vi "HGCalSensorTesting.vi"() -> ()   [LabVIEW 2016]
uses:
  <vilib>/Utility/file.llb/Read Delimited Spreadsheet (string).vi
  <vilib>/Utility/file.llb/Read Delimited Spreadsheet (DBL).vi
  <vilib>/Utility/file.llb/Read Delimited Spreadsheet (I64).vi
  <vilib>/Utility/file.llb/Write Delimited Spreadsheet (string).vi
panel:
  in  "Channel to Monitor:":i32
  out "XY Graph 3":cluster{"Y":dbl[], "Y":dbl[]}[](graph)
  in  "Switch Delay (s)":dbl format="%#_13g"
  in  "Voltage Delay (s)":dbl format="%#_13g"
  out "XY Graph 2":cluster{"Y":dbl[], "Y":dbl[]}[](graph)
  out "XY Graph":cluster{"Y":dbl[], "Y":dbl[]}[](graph)
  out "Errors":errorcluster
  in  "Measurement Data":string[][](table)
  in  "Select Measurement Type":enum16{"I-V", "C-V", "Cij"}(ring)
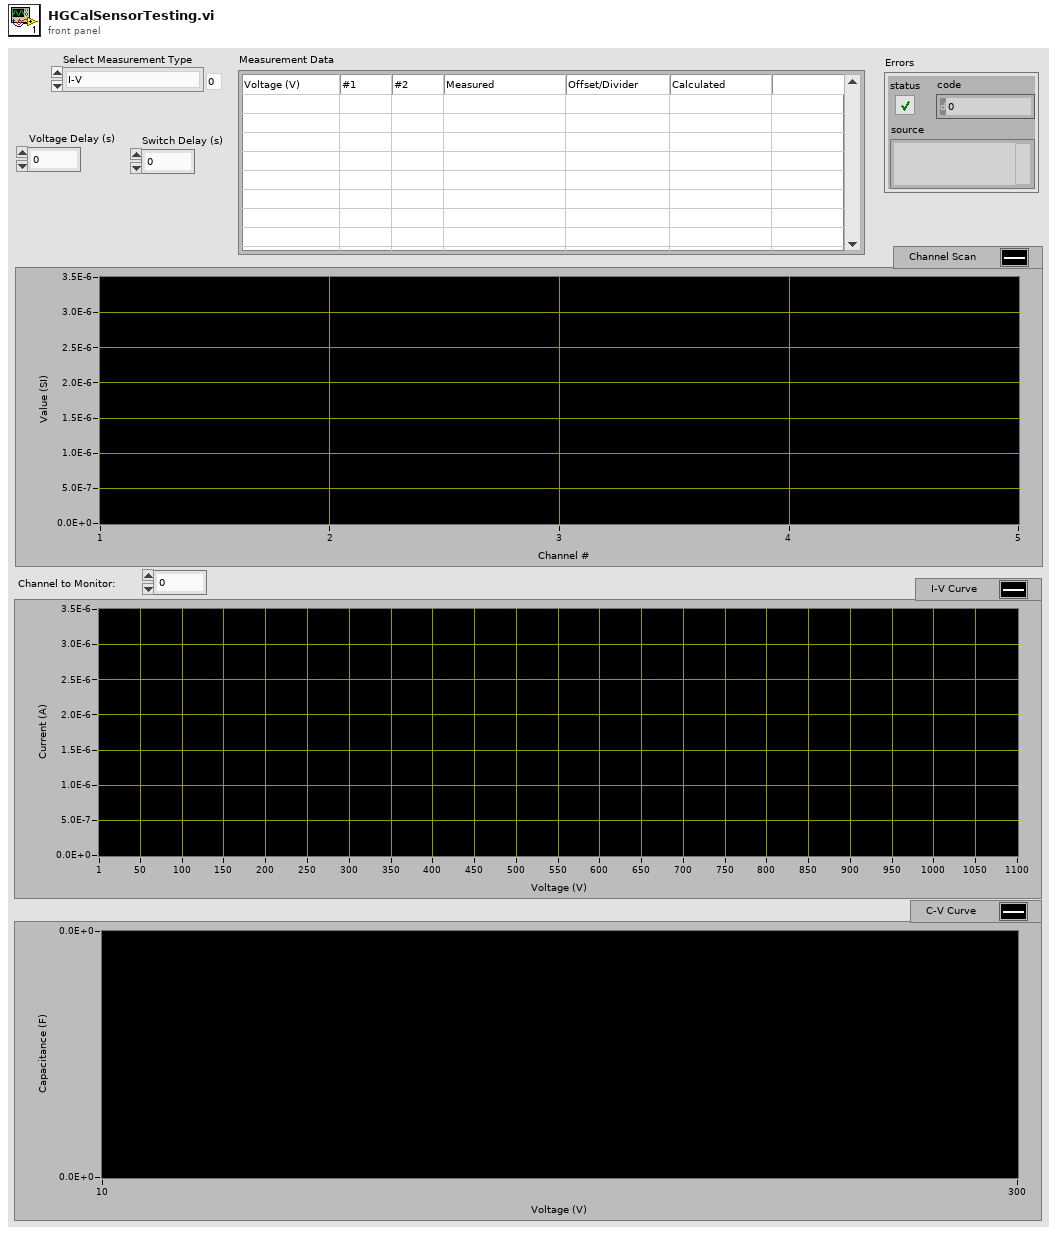
[diagram p1: front panel]
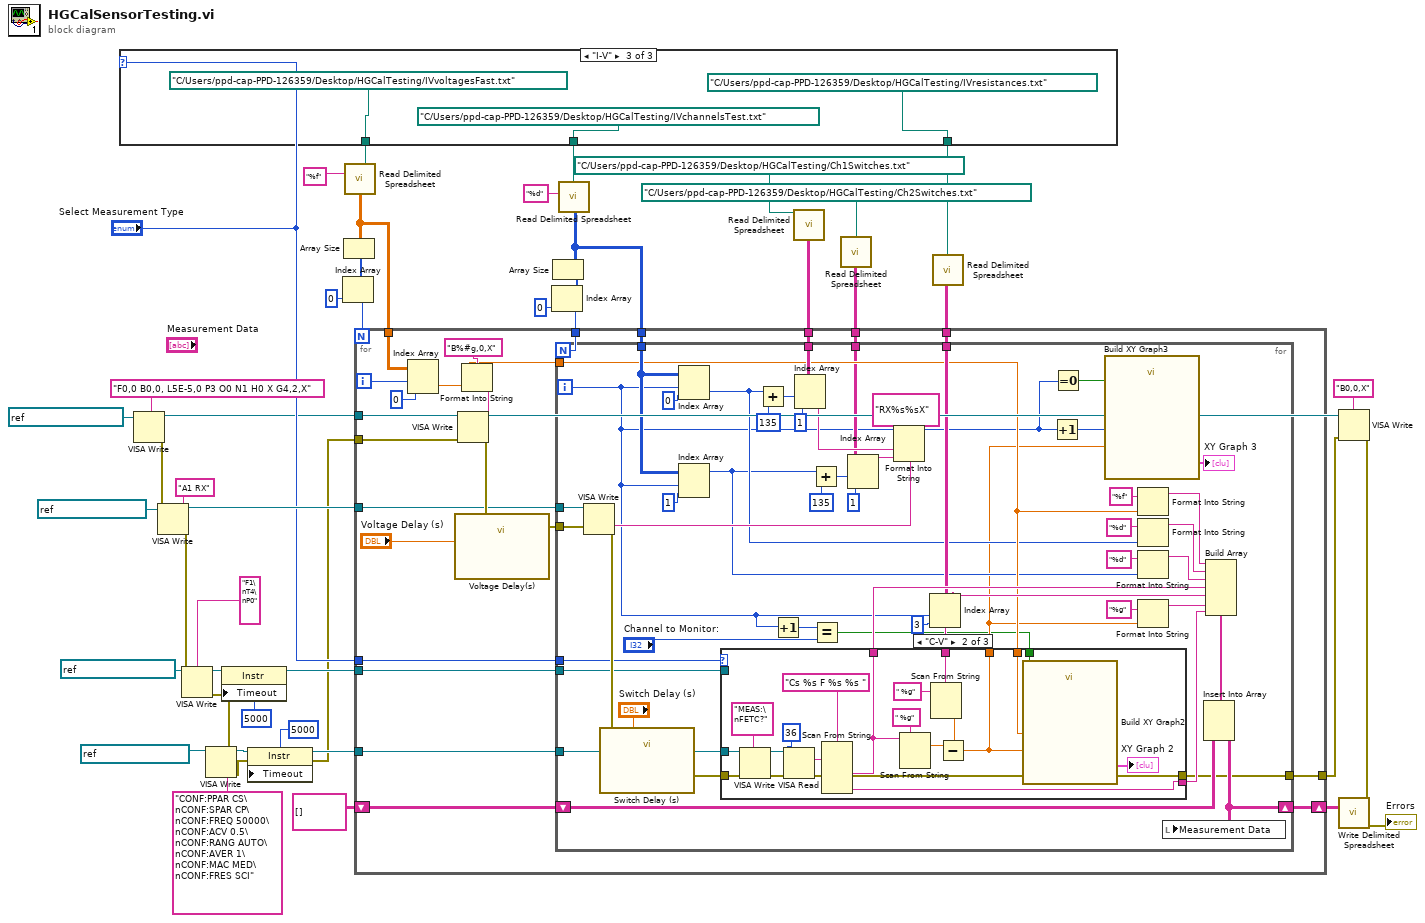
[diagram p0: block diagram]
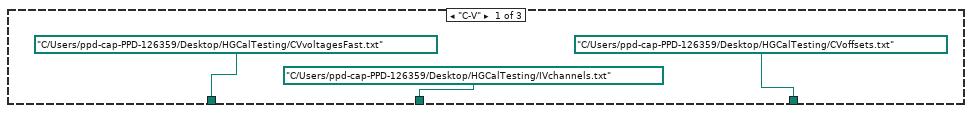
[diagram p2: hidden frame]
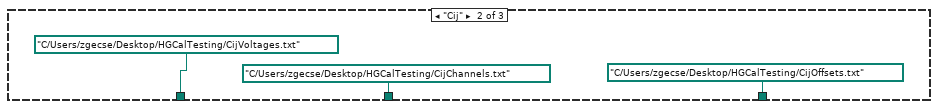
[diagram p3: hidden frame]
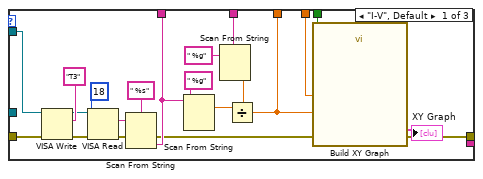
[diagram p4: hidden frame]
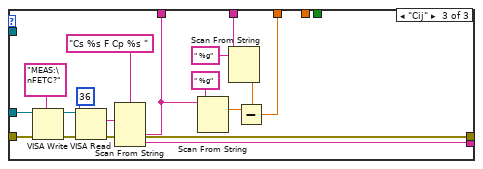
[diagram p5: hidden frame]
diagram:
  n1 = case shown="\"I-V\"" "Select Measurement Type" {
    tunnel: [path "C:/Users/ppd-cap-PPD-126359/Desktop/HGCalTesting/CVvoltagesFast.txt" ("file path (dialog if empty)") path "C:/Users/zgecse/Desktop/HGCalTesting/CijVoltages.txt" ("file path (dialog if empty)") path "C:/Users/ppd-cap-PPD-126359/Desktop/HGCalTesting/IVvoltagesFast.txt" ("file path (dialog if empty)")] -> w37
    tunnel: [path "C:/Users/ppd-cap-PPD-126359/Desktop/HGCalTesting/IVchannels.txt" ("file path (dialog if empty)") path "C:/Users/zgecse/Desktop/HGCalTesting/CijChannels.txt" ("file path (dialog if empty)") path "C:/Users/ppd-cap-PPD-126359/Desktop/HGCalTesting/IVchannelsTest.txt" ("file path (dialog if empty)")] -> w35
    tunnel: [path "C:/Users/ppd-cap-PPD-126359/Desktop/HGCalTesting/CVoffsets.txt" ("file path (dialog if empty)") path "C:/Users/zgecse/Desktop/HGCalTesting/CijOffsets.txt" ("file path (dialog if empty)") path "C:/Users/ppd-cap-PPD-126359/Desktop/HGCalTesting/IVresistances.txt" ("file path (dialog if empty)")] -> w20
    frame "C-V" {
    }
    frame "Cij" {
    }
    frame "I-V" {
    }
  }
  n2 = VISA Write(VISA resource name=refnum<visa-resource-name> "GPIB1::10::INSTR" ("K237 VISA"), write buffer="F0,0 B0,0, L5E-5,0 P3 O0 N1 H0 X G4,2,X" ("F0,0X B%f,0,X L%f,0X P3X O0X")) -> (VISA resource name out=w5:refnum<visa-resource-name>, error out=w43:errorcluster)  [unwired: 1 in, 1 out]
  n3 = VISA Write(VISA resource name=refnum<visa-resource-name> "GPIB1::3::INSTR" ("K706 VISA"), write buffer="A1 RX" ("F0,0X B%f,0,X L%f,0X P3X O0X"), error in (no error)=w43) -> (VISA resource name out=w33:refnum<visa-resource-name>, error out=w38:errorcluster)  [unwired: 1 out]
  n4 = VISA Write(VISA resource name=refnum<visa-resource-name> "GPIB1::22::INSTR" ("K706 VISA"), write buffer="F1\nT4\nP0" ("F0,0X B%f,0,X L%f,0X P3X O0X"), error in (no error)=w38) -> (VISA resource name out=w18:refnum<visa-resource-name>, error out=w16:errorcluster)  [unwired: 1 out]
  n5 = property class="Instr"(reference=w18, error in=w16, "Timeout"=u32 5000 ("General Settings:Timeout Value")) -> (reference out=w17:refnum<visa-resource-name>, error out=w15:errorcluster)
  n6 = VISA Write(VISA resource name=refnum<visa-resource-name> "GPIB1::4::INSTR" ("K706 VISA"), write buffer="CONF:PPAR CS\nCONF:SPAR CP\nCONF:FREQ 50000\nCONF:ACV 0.5\nCONF:RANG AUTO\nCONF:AVER 1\nCONF:MAC MED\nCONF:FRES SCI" ("F0,0X B%f,0,X L%f,0X P3X O0X"), error in (no error)=w15) -> (VISA resource name out=w12:refnum<visa-resource-name>, error out=w10:errorcluster)  [unwired: 1 out]
  n7 = property class="Instr"(reference=w12, error in=w10, "Timeout"=u32 5000 ("General Settings:Timeout Value")) -> (reference out=w11:refnum<visa-resource-name>, error out=w9:errorcluster)
  n8 = call-poly <vilib>:"Read Delimited Spreadsheet.vi"("file path (dialog if empty)"=w37, "format (%.3f)"="%f") -> ("all rows"=w23:dbl[][])  [unwired: 8 in, 5 out]
  n9 = Array Size(array=w23) -> (size(s)=w25:i32[])
  n10 = Index Array(array=w25, index=0) -> (element=w24:i32)
  n11 = call-poly <vilib>:"Read Delimited Spreadsheet.vi"("file path (dialog if empty)"=w35, "format (%d)"="%d" ("format (%.3f)")) -> ("all rows"=w30:i64[][])  [unwired: 8 in, 5 out]
  n12 = Array Size(array=w30) -> (size(s)=w32:i32[])
  n13 = Index Array(array=w32, index=0) -> (element=w6:i32)
  n14 = call-poly <vilib>:"Read Delimited Spreadsheet.vi"("file path (dialog if empty)"=path "C:/Users/ppd-cap-PPD-126359/Desktop/HGCalTesting/Ch1Switches.txt") -> ("all rows"=w29:string[][])  [unwired: 9 in, 5 out]
  n15 = call-poly <vilib>:"Read Delimited Spreadsheet.vi"("file path (dialog if empty)"=path "C:/Users/ppd-cap-PPD-126359/Desktop/HGCalTesting/Ch2Switches.txt") -> ("all rows"=w7:string[][])  [unwired: 9 in, 5 out]
  n16 = call-poly <vilib>:"Read Delimited Spreadsheet.vi"("file path (dialog if empty)"=w20) -> ("all rows"=w19:string[][])  [unwired: 9 in, 5 out]
  n17 = for {
    N: w24 -> [_]
    tunnel: w23 -> [w77]
    tunnel: w5 -> [w73]
    tunnel: w9 -> [w71]
    tunnel: w30 -> [w70]
    tunnel: w6 -> [w69]
    tunnel: w33 -> [w68]
    tunnel: w29 -> [w66]
    tunnel: w17 -> [w65]
    shift-right: [w63] -> w27
    shift-left: string[][] [] -> [w64]
    tunnel: "Select Measurement Type" -> [w61]
    tunnel: w11 -> [w60]
    tunnel: w19 -> [w59]
    tunnel: w7 -> [w58]
    tunnel: [w57] -> w2
    i -> [w78]
    n18 = Index Array(array=w77, index (row)=w78, index (col)=0 ("disabled index (col)")) -> (element=w62:dbl)
    n19 = Format Into String(format string="B%#g,0,X" ("F0,0X B%f,0,X L%f,0X P3X O0X"), w62) -> (resulting string=w72:string)  [unwired: 2 in, 1 out]
    n20 = VISA Write(VISA resource name=w73, write buffer=w72, error in (no error)=w71) -> (error out=w76:errorcluster)  [unwired: 2 out]
    n21 = call "Voltage Delay(s)"("error in (no error)"=w76, "Delay Time (s)"="Voltage Delay (s)") -> ("error out"=w67:errorcluster)  [unwired: 9 in]
    n22 = for {
      N: w69 -> [_]
      tunnel: w70 -> [w127]
      tunnel: w68 -> [w126]
      tunnel: w67 -> [w125]
      tunnel: w66 -> [w123]
      tunnel: w65 -> [w120]
      shift-right: [w117] -> w63
      shift-left: w64 -> [w118]
      tunnel: w62 -> [w102]
      tunnel: w61 -> [w108]
      tunnel: w60 -> [w107]
      tunnel: w59 -> [w104]
      tunnel: w58 -> [w94]
      tunnel: [w80] -> w57
      i -> [w82]
      n23 = Index Array(array=w127, index (row)=w82, index (col)=0 ("disabled index (col)")) -> (element=w100:i64)
      n24 = Index Array(array=w127, index (row)=w82, index (col)=1 ("disabled index (col)")) -> (element=w92:i64)
      n25 = Add(x=w100, y=i64 135) -> (x+y=w101:i64)
      n26 = Increment(x=w82) -> (x+1=w85:i32)
      n27 = Index Array(array=w123, index (row)=w101, index (col)=1 ("disabled index (col)")) -> (element=w98:string)
      n28 = Add(x=w92, y=i64 135) -> (x+y=w96:i64)
      n29 = Equal?(x=w85, y="Channel to Monitor:") -> (x = y?=w86:bool)
      n30 = Index Array(array=w94, index (row)=w96, index (col)=1 ("disabled index (col)")) -> (element=w93:string)
      n31 = Format Into String(format string="RX%s%sX", w98, w93) -> (resulting string=w106:string)  [unwired: 2 in, 1 out]
      n32 = VISA Write(VISA resource name=w126, write buffer=w106, error in (no error)=w125) -> (error out=w121:errorcluster)  [unwired: 2 out]
      n33 = call "Switch Delay (s)"("error in (no error)"=w121, "Delay Time (s)"="Switch Delay (s)") -> ("error out"=w119:errorcluster)  [unwired: 9 in]
      n34 = Index Array(array=w104, index (row)=w82, index (col)=3 ("disabled index (col)")) -> (element=w103:string)
      n35 = case shown="\"C-V\"" w108 {
        tunnel: w120 -> [w139 _ _]
        tunnel: w119 -> [w137 w166 w183]
        tunnel: [w143 w157 w174] -> w109
        tunnel: w107 -> [_ w165 w182]
        tunnel: w103 -> [w146 w156 w173]
        tunnel: w102 -> [w134 w154 _]
        tunnel: [w133 w153 w172] -> w88
        tunnel: w86 -> [w132 w152 _]
        tunnel: [_ w151 w171] -> w81
        tunnel: [w131 w150 w170] -> w80
        frame "I-V", Default {
          n36 = VISA Write(VISA resource name=w139, write buffer="T3", error in (no error)=w137) -> (VISA resource name out=w138:refnum<visa-resource-name>, error out=w136:errorcluster)  [unwired: 1 out]
          n37 = VISA Read(VISA resource name=w138, byte count=u32 18 ("HP read count"), error in (no error)=w136) -> (read buffer=w147:string, error out=w131:errorcluster)  [unwired: 2 out]
          n38 = Scan From String(format string=" %s", input string=w147) -> (output 1=w143:string)  [unwired: 3 in, 3 out]
          n39 = Scan From String(format string=" %g", input string=w143) -> (output 1=w142:dbl)  [unwired: 3 in, 3 out]
          n40 = Scan From String(format string=" %g", input string=w146) -> (output 1=w141:dbl)  [unwired: 3 in, 3 out]
          n41 = Divide(x=w142, y=w141) -> (x/y=w133:dbl)
          n42 = call "Build XY Graph"("Enable"=w132, "Y Input"=w133, "X Input"=w134) -> ("XY Graph"=→"XY Graph":cluster{"X":dbl[], "Y":dbl[]}[])  [unwired: 7 in, 1 out]
        }
        frame "C-V" {
          n43 = VISA Write(VISA resource name=w165, write buffer="MEAS:\nFETC?", error in (no error)=w166) -> (VISA resource name out=w163:refnum<visa-resource-name>, error out=w164:errorcluster)  [unwired: 1 out]
          n44 = VISA Read(VISA resource name=w163, byte count=u32 36 ("byte count 2"), error in (no error)=w164) -> (read buffer=w162:string, error out=w150:errorcluster)  [unwired: 2 out]
          n45 = Scan From String(format string="Cs %s F %s %s ", input string=w162) -> (output 1=w157:string, output 3=w151:string)  [unwired: 6 in, 3 out]
          n46 = Scan From String(format string=" %g", input string=w157) -> (output 1=w160:dbl)  [unwired: 3 in, 3 out]
          n47 = Scan From String(format string=" %g", input string=w156) -> (output 1=w161:dbl)  [unwired: 3 in, 3 out]
          n48 = Subtract(x=w160, y=w161) -> (x-y=w153:dbl)
          n49 = call "Build XY Graph2"("Enable"=w152, "Y Input"=w153, "X Input"=w154) -> ("XY Graph"=→"XY Graph 2":cluster{"X":dbl[], "Y":dbl[]}[])  [unwired: 7 in, 1 out]
        }
        frame "Cij" {
          n50 = VISA Write(VISA resource name=w182, write buffer="MEAS:\nFETC?", error in (no error)=w183) -> (VISA resource name out=w180:refnum<visa-resource-name>, error out=w181:errorcluster)  [unwired: 1 out]
          n51 = VISA Read(VISA resource name=w180, byte count=u32 36 ("byte count 2"), error in (no error)=w181) -> (read buffer=w179:string, error out=w170:errorcluster)  [unwired: 2 out]
          n52 = Scan From String(format string="Cs %s F Cp %s ", input string=w179) -> (output 1=w174:string, output 2=w171:string)  [unwired: 4 in, 3 out]
          n53 = Scan From String(format string=" %g", input string=w174) -> (output 1=w176:dbl)  [unwired: 3 in, 3 out]
          n54 = Scan From String(format string=" %g", input string=w173) -> (output 1=w175:dbl)  [unwired: 3 in, 3 out]
          n55 = Subtract(x=w176, y=w175) -> (x-y=w172:dbl)
        }
      }
      n56 = Increment(x=w82) -> (x+1=w83:i32)
      n57 = Equal To 0?(x=w82) -> (x = 0?=w84:bool)
      n58 = call "Build XY Graph3"("Reset"=w84, "Y Input"=w88, "X Input"=w83) -> ("XY Graph"=→"XY Graph 3":cluster{"X":dbl[], "Y":dbl[]}[])  [unwired: 7 in, 1 out]
      n59 = Format Into String(format string="%f", w102) -> (resulting string=w113:string)  [unwired: 2 in, 1 out]
      n60 = Format Into String(format string="%d", w100) -> (resulting string=w112:string)  [unwired: 2 in, 1 out]
      n61 = Format Into String(format string="%d", w92) -> (resulting string=w111:string)  [unwired: 2 in, 1 out]
      n62 = Format Into String(format string="%g", w88) -> (resulting string=w90:string)  [unwired: 2 in, 1 out]
      n63 = Build Array(w113, w112, w111, w109, w103, w90, w81) -> (w110:string[])
      n64 = Insert Into Array(array=w118, new element=w110) -> (w117:string[][])  [unwired: 2 in]
      n65 = local write "Measurement Data"(w117) -> ()
    }
  }
  n66 = VISA Write(VISA resource name=w5, write buffer="B0,0,X" ("F0,0X B%f,0,X L%f,0X P3X O0X"), error in (no error)=w2) -> (error out=w1:errorcluster)  [unwired: 2 out]
  n67 = call-poly <vilib>:"Write Delimited Spreadsheet.vi"("2D data"=w27, "error in (no error)"=w1) -> ("error out"=→"Errors":errorcluster)  [unwired: 12 in, 1 out]
